vi "picoquant_initialize_acq_mode.vi"(8 "error in (no error)":errorcluster, 11 "picoquant_generic in":refnum<class "picoquant_generic.lvclass">) -> (0 "error out":errorcluster, 3 "picoquant_generic out":refnum<class "picoquant_generic.lvclass">)   [LabVIEW 2015, in "picoquant_generic.lvclass"]
uses:
  picoquant_generic.lvclass
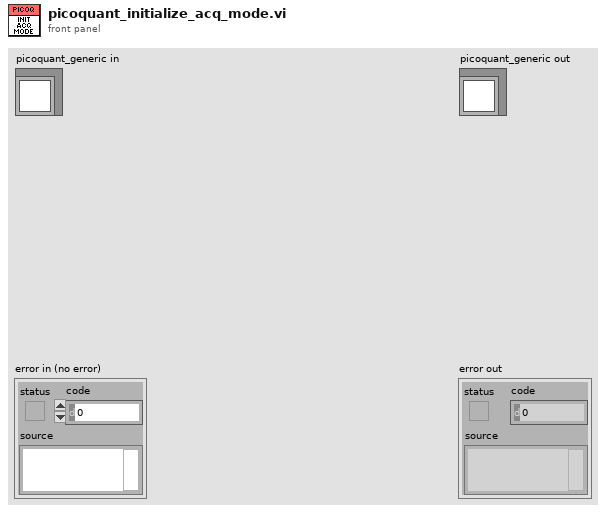
[diagram p1: front panel]
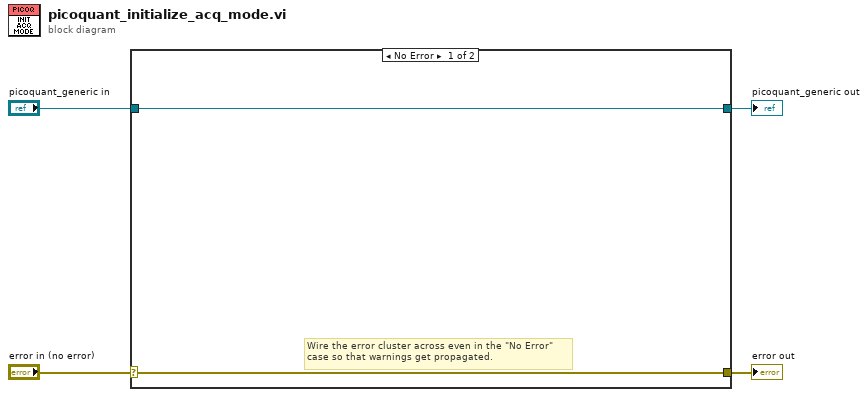
[diagram p0: block diagram]
diagram:
  n1 = case shown="No Error" "error in (no error)" {
    selector: "error in (no error)" -> [w5 w8]
    tunnel: [w5 w8] -> w3
    tunnel: [w6 w7] -> w1
    tunnel: "picoquant_generic in" -> [w6 w7]
    frame No Error {
      # "Wire the error cluster across even in the \"No Error\"\ncase so that warnings get propagated."
    }
    frame Error {
    }
  }
  "error out" <- w3
  "picoquant_generic out" <- w1
